vi "Draw.vi"(1 "Center position in":refnum<class "Vector2.lvclass">, 2 "Picture in":picture, 3 "Simulation Object in":refnum<class "SimulationObject.lvclass">) -> (0 "Picture out":picture)   [LabVIEW 2022 SP3, in "DrawComponent.lvclass"]
uses:
  DrawComponent.lvclass
  Math/Vector2/Vector2.lvclass
  SimulationObject/SimulationObject.lvclass
  Transform/Transform.lvclass
  Shapes/Shapeable/Shapeable.lvclass
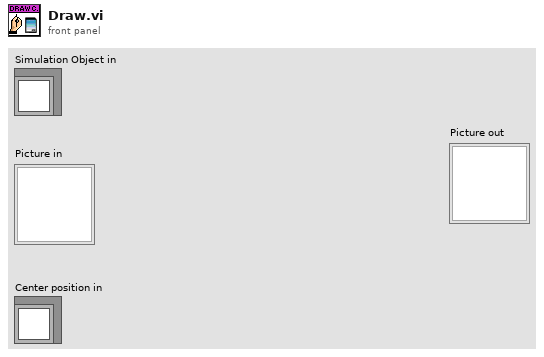
[diagram p1: front panel]
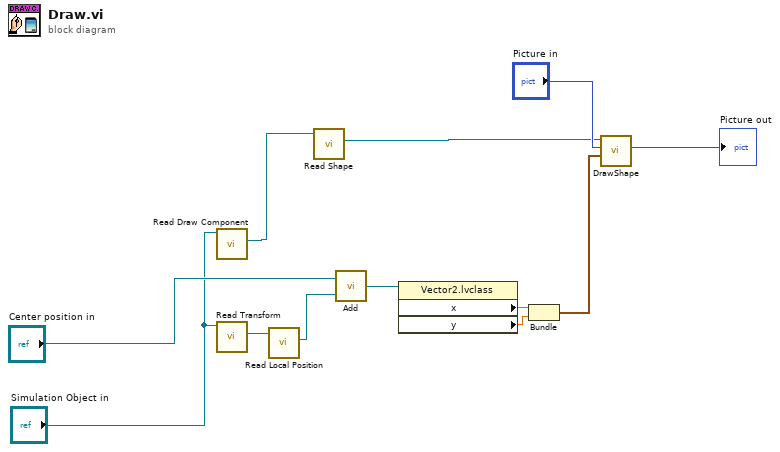
[diagram p0: block diagram]
diagram:
  n1 = call "Read Draw Component.vi"("SimulationObject in"="Simulation Object in") -> ("Draw Component out"=w2:refnum<class "DrawComponent.lvclass">)  [unwired: 8 in, 2 out]
  n2 = call "Read Transform.vi"("SimulationObject in"="Simulation Object in") -> ("Transform out"=w9:refnum<class "Transform.lvclass">)  [unwired: 8 in, 2 out]
  n3 = call "Read Local Position.vi"("Transform in"=w9) -> ("Local Position out"=w8:refnum<class "Vector2.lvclass">)  [unwired: 8 in, 2 out]
  n4 = call "Read Shape.vi"("DrawComponent in"=w2) -> ("Shape"=w3:refnum<class "Shapeable.lvclass">)  [unwired: 8 in, 2 out]
  n5 = call "Add.vi"("Vec2 b in"=w8, "Vec2 a in"="Center position in") -> ("Vec2 out"=w12:refnum<class "Vector2.lvclass">)
  n6 = property class="Vector2.lvclass"(reference=w12) -> ("x"=w11:sgl, "y"=w10:sgl)  [unwired: 1 in, 2 out]
  n7 = Bundle("x"=w11, "y"=w10) -> (w1:cluster{"x":sgl, "y":sgl})  [unwired: 1 in]
  n8 = call-dynamic "DrawShape.vi"("Center Position in"=w1, "Picture in"="Picture in", "Shapeable in"=w3) -> ("Picture out"=→"Picture out":picture)  [unwired: 6 in, 2 out]
